vi "global_act_eje_edif.vi"() -> ()   [LabVIEW 2017]
panel:
  out "act_prog_edif":bool
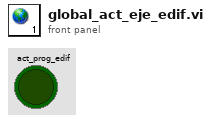
[diagram p1: front panel]
diagram:
